vi "ActuatorSetup_HORNDOWN_1000.vi"() -> ()   [LabVIEW 2017]
uses:
  Generic_Common/WeldAutomation/Global_Variable_Status_Indicator.vi
panel:
  out "Pre part contanct in inch":dbl
  out "Pre Part Contanct distance in mm pre":dbl
  out "Absolute distance in inch":dbl
  out "Absolute distance in mm":dbl
  out "#Iterations:":dbl format="%-#1.6g"
  out "Welding Progress":u8(slide) scale=0.0..100.0
  out "Test Result":picture
  out "Performance Graph":cluster{dbl, u32}[](graph)
  # "Instructions:\n1. Make sure Ethernet cable from SC board connected to Laptop, \n2. Type netstat in command pompt to cross verify, SC port connection is established \n3. Then run the VI, press palm button first time button for actuator setup FPC will be perfomed\n4. Again press palm button to perform welding, second time onward welding will be perfomed\n5, To edit local_config.ini file to change the recipe parameters."
  # "Test execution sequence : \n1. Read SC, PC_AC parameters from INI file\n2. Send command to BL\n    a. MessageID_SC + Length (SC parameters) + SC parameters\n      b. MessageID_PC_AC  + Length (PC_AC parameters) + PC_AC parameters\n3. Receive response from BL after sending recipe parameters\n      c. ResponseID + Message \n4. Press palm button using USB6008 device\n5. Report Generation and Log generation"
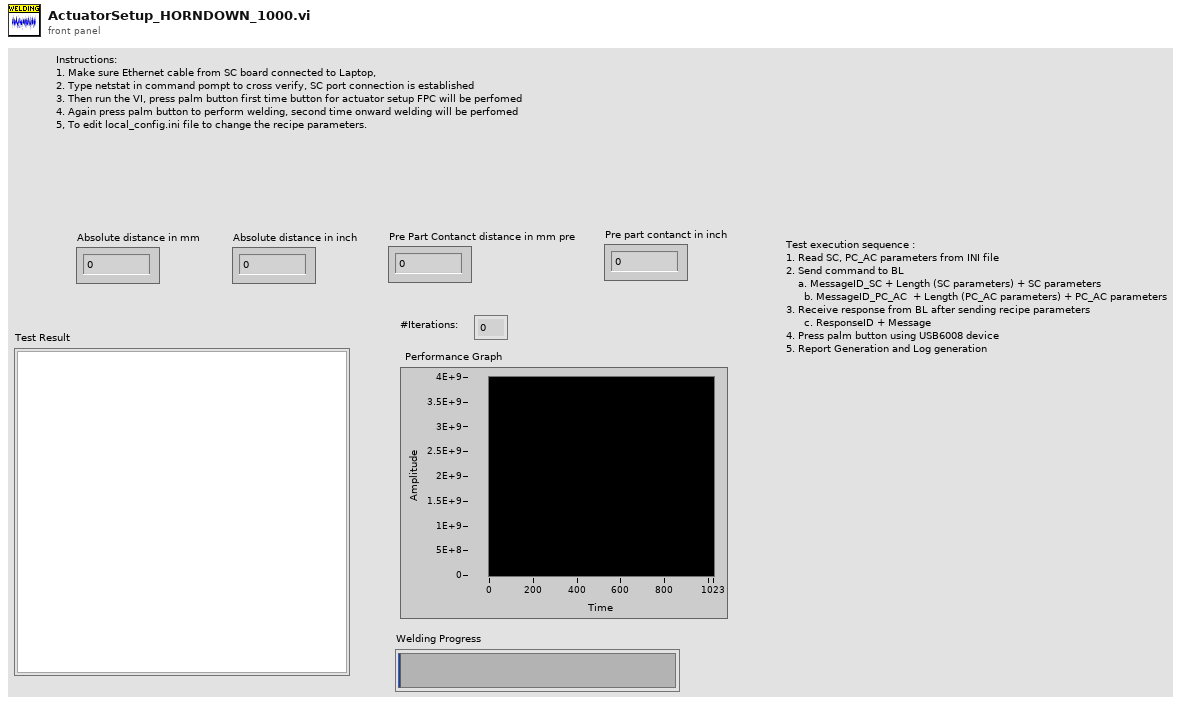
[diagram p1: front panel]
types:
  T1 = enum16{"open", "replace", "create", "open or create", "replace or create", "replace or create with confirmation"}
  T2 = cluster{"[0]":string, "[1]":string, "[2]":string, "[3]":string, "[4]":string, "[5]":string, "[6]":string, "[7]":string, "[8]":string}
  T3 = cluster{"Socket_IP_Address":string, "Socket_Port_Number":u16, "Global_ReportPath":path}
  T4 = cluster{"Iterations":u64, "DelayBetweenIterations":u32, "Time out":u32, "Message ID":i32, "Message Lenght":i32, "Response ID":i32, "Type of operation":i32, "Time stamp":string, "Test suite":string, "Report Path":path, "FW Version Path":path}
  T5 = typedef "imagedata.ctl" = cluster{"image type":i32, "image depth":i32, "image":u8[], "mask":u8[], "colors":u32[], "Rectangle":cluster{"left":i16, "top":i16, "right":i16, "bottom":i16}}
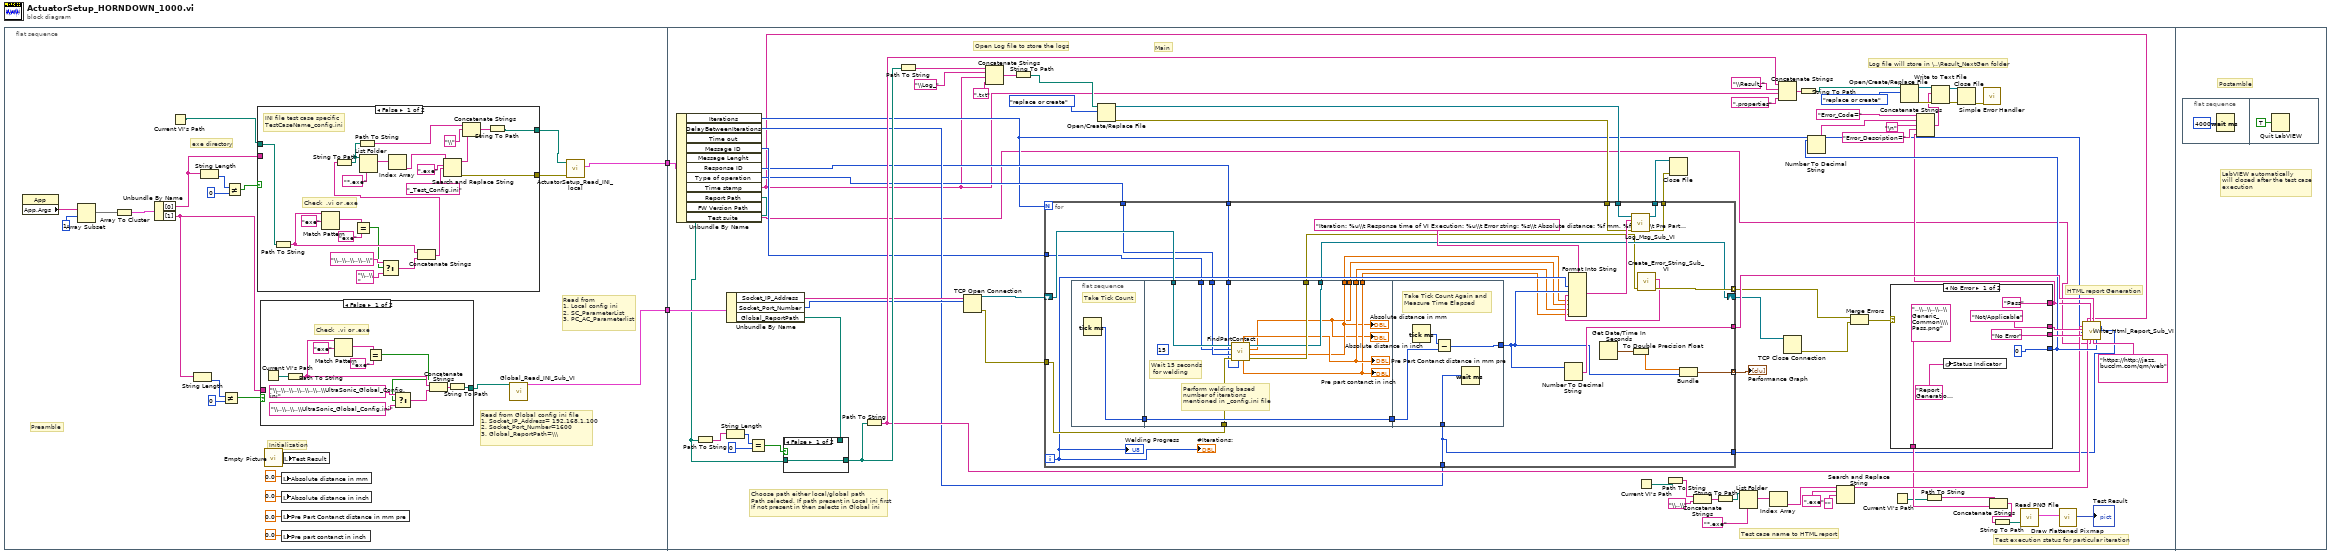
[diagram p0: block diagram]
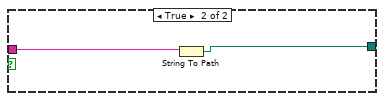
[diagram p2: hidden frame]
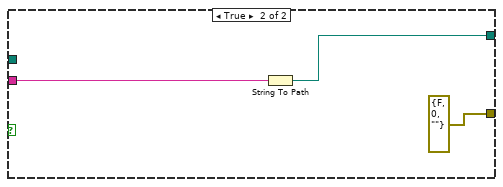
[diagram p3: hidden frame]
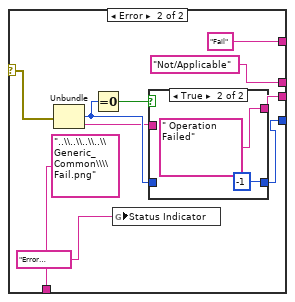
[diagram p5: hidden frame]
diagram:
  n1 = flat-sequence {
    tunnel: [w12] -> w2
    tunnel: [w8] -> w1
    tunnel: w2 -> [w86]
    tunnel: w1 -> [w71]
    frame #0 {
      # "Initialization"
      # "exe directory"
      # "Read from Global config ini file\n1. Socket_IP_Address= 192.168.1.100\n2. Socket_Port_Number=1600\n3. Global_ReportPath=\\\\\\"
      # "Read from\n1. Local config ini\n2. SC_ParameterList\n3. PC_AC_Parameterlist"
      # "Preamble"
      n2 = property class="App"() -> ("App.Args"=w14:string[])  [unwired: 2 in, 2 out]
      n3 = Array Subset "Array Subset"(array=w14, index=1) -> (w15:string[])  [unwired: 1 in]
      n4 = Array To Cluster(array=w15) -> (cluster=w16:T2)
      n5 = Unbundle By Name "Unbundle By Name"(w16) -> ("[0]"=w20:string, "[1]"=w23:string)
      n6 = Current VI's Path() -> (path=w11:path)
      n7 = String Length(string=w23) -> (length=w24:i32)
      n8 = String Length(string=w20) -> (length=w17:i32)
      n9 = Not Equal?(x=w24, y=0) -> (x != y?=w22:bool)
      n10 = Not Equal?(x=w17, y=0) -> (x != y?=w19:bool)
      n11 = case shown="False" w19 {
        tunnel: w20 -> [_ w63]
        tunnel: [w52 w62] -> w10
        tunnel: [w51 errorcluster {"status"=FALSE, "code"=0, "source"=""} ("error out")] -> w9
        tunnel: w11 -> [w40 _]
        frame False {
          # "Check  .vi or .exe"
          # "INI file test case specific\nTestCaseName_config.ini"
          n12 = Path To String(path=w40) -> (string=w45:string)
          n13 = Match Pattern(string=w45, regular expression="exe") -> (match substring=w44:string)  [unwired: 1 in, 3 out]
          n14 = Equal?(x=w44, y="exe") -> (x = y?=w42:bool)
          n15 = Select(t="\\..\\..\\..\\..\\" ("string"), s=w42, f="\\..\\" ("string")) -> (s? t:f=w46:string)
          n16 = Concatenate Strings(w45, w46) -> (w39:string)
          n17 = String To Path(string=w39) -> (path=w50:path)
          n18 = Path To String(path=w50) -> (string=w49:string)
          n19 = List Folder(path=w50, pattern="*.exe") -> (filenames=w54:string[])  [unwired: 2 in, 3 out]
          n20 = Index Array(array=w54) -> (element=w53:string)  [unwired: 1 in]
          n21 = Search and Replace String(input string=w53, search string=".exe", replace string="_Test_Config.ini" ("replace string (\"\")")) -> (result string=w58:string, error out=w51:errorcluster)  [unwired: 5 in, 2 out]
          n22 = Concatenate Strings(w49, "\\" ("string"), w58) -> (w56:string)
          n23 = String To Path(string=w56) -> (path=w52:path)
        }
        frame True {
          n24 = String To Path(string=w63) -> (path=w62:path)
        }
      }
      n25 = case shown="False" w22 {
        tunnel: [w35 w38] -> w25
        tunnel: w23 -> [_ w37]
        frame False {
          # "Check  .vi or .exe"
          n26 = Current VI's Path() -> (path=w27:path)
          n27 = Path To String(path=w27) -> (string=w31:string)
          n28 = Match Pattern(string=w31, regular expression="exe") -> (match substring=w30:string)  [unwired: 1 in, 3 out]
          n29 = Equal?(x=w30, y="exe") -> (x = y?=w28:bool)
          n30 = Select(t="\\..\\..\\..\\..\\..\\..\\UltraSonic_Global_Config.ini" ("string"), s=w28, f="\\..\\..\\..\\UltraSonic_Global_Config.ini" ("string")) -> (s? t:f=w32:string)
          n31 = Concatenate Strings(w31, w32) -> (w36:string)
          n32 = String To Path(string=w36) -> (path=w35:path)
        }
        frame True {
          n33 = String To Path(string=w37) -> (path=w38:path)
        }
      }
      n34 = call "Empty Picture"() -> ("empty picture"=w3:picture)
      n35 = local write "Absolute distance in mm"(0.0) -> ()
      n36 = local write "Absolute distance in inch"(0.0) -> ()
      n37 = local write "Pre Part Contanct distance in mm pre"(0.0) -> ()
      n38 = local write "Pre part contanct in inch"(0.0) -> ()
      n39 = local write "Test Result"(w3) -> ()
      n40 = call "Global_Read_INI_Sub_VI.vi"("Config File Path"=w25) -> ("output cluster"=w12:T3)  [unwired: 14 in]
      n41 = call "ActuatorSetup_Read_INI_local.vi"("Error In"=w9, "Config File Path"=w10) -> ("Actuator setup Parameters"=w8:T4)  [unwired: 8 in, 1 out]
    }
    frame #1 {
      # "Open Log file to store the logs"
      # "HTML report Generation"
      # "Log file will store in \\..\\Result_NextGen folder"
      # "Test execution status for particular iteration"
      # "Test case name to HTML report"
      # "Choose path either local/global path\nPath selected, If path present in Local ini first\nIf not present in then selects in Global ini"
      # "Main"
      n42 = Unbundle By Name(w71) -> ("Iterations"=w67:u64, "DelayBetweenIterations"=w74:u32, "Message ID"=w70:i32, "Response ID"=w69:i32, "Type of operation"=w68:i32, "Time stamp"=w65:string, "Report Path"=w72:path, "Test suite"=w66:string)  [unwired: 3 out]
      n43 = Path To String(path=w72) -> (string=w73:string)
      n44 = String Length(string=w73) -> (length=w129:i32)
      n45 = Unbundle By Name(w86) -> ("Socket_IP_Address"=w83:string, "Socket_Port_Number"=w82:u16, "Global_ReportPath"=w85:path)
      n46 = Equal?(x=w129, y=0) -> (x = y?=w127:bool)
      n47 = case shown="False" w127 {
        tunnel: w85 -> [_ w141]
        tunnel: [w140 w141] -> w126
        tunnel: w72 -> [w140 _]
        frame False {
        }
        frame True {
        }
      }
      n48 = Path To String(path=w126) -> (string=w103:string)
      n49 = Path To String(path=w126) -> (string=w131:string)
      n50 = TCP Open Connection(address=w83, remote port or service name=w82) -> (connection ID=w79:refnum<k5>, error out=w81:errorcluster)  [unwired: 3 in]
      n51 = Concatenate Strings(w131, "\\Log_" ("string"), w65, ".txt" ("string")) -> (w134:string)
      n52 = String To Path(string=w134) -> (path=w133:path)
      n53 = Open/Create/Replace File(file path (use dialog)=w133, operation (0:open)=T1."replace or create") -> (refnum out=w104:refnum<file>, error out=w107:errorcluster)  [unwired: 1 in, 4 out]
      n54 = for {
        N: w67 -> [_]
        tunnel: [w168] -> w137
        tunnel: w104 -> [w162]
        tunnel: [w161] -> w106
        tunnel: [w159] -> w105
        tunnel: [w164] -> w135 mode=indexing
        tunnel: w107 -> [w160]
        tunnel: [w157] -> w102 mode=indexing
        tunnel: w81 -> [w155]
        shift-right: [w152] -> w80
        shift-left: w79 -> [w154]
        tunnel: w74 -> [w142]
        tunnel: w68 -> [w145]
        tunnel: w70 -> [w144]
        tunnel: w69 -> [w143]
        tunnel: [w142] -> w64
        i -> [w153]
        n55 = flat-sequence {
          tunnel: [w170] -> w169
          tunnel: [w182] -> w151
          tunnel: w169 -> [w182]
          tunnel: w155 -> [w180]
          tunnel: w154 -> [w181]
          tunnel: [w178] -> w152
          tunnel: [w179] -> w150
          tunnel: [w172] -> w149
          tunnel: [w171] -> w148
          tunnel: [w177] -> w147
          tunnel: [w176] -> w146
          tunnel: w145 -> [w175]
          tunnel: w144 -> [w174]
          tunnel: w143 -> [w173]
          tunnel: w151 -> [w186]
          tunnel: [w184] -> w158
          tunnel: w142 -> [w183]
          frame #0 {
            # "Take Tick Count"
            n56 = Tick Count (ms)() -> (millisecond timer value=w170:u32)
          }
          frame #1 {
            (unwired) 15
            # "Wait 15 seconds\n for welding"
            # "Perform welding based \nnumber of iterations\nmentioned in _config.ini file"
            n57 = call "FindPartContact.vi"("Response actuator"=w173, "Error In"=w180, "Type of operation"=w175, "Actuator command"=w174, "connection ID"=w181) -> ("Error Out"=w179:errorcluster, "Absolute distance mm"=w172:dbl, "Absolute distance inch"=w171:dbl, "connection ID out"=w178:refnum<k5>, "Pre Part contact inch"=w176:dbl, "Pre Part Contact mm"=w177:dbl)  [unwired: 1 in]
            "Absolute distance in mm" <- w172
            "Absolute distance in inch" <- w171
            "Pre Part Contanct distance in mm pre" <- w177
            "Pre part contanct in inch" <- w176
          }
          frame #2 {
            # "Take Tick Count Again and Measure Time Elapsed"
            n58 = Tick Count (ms)() -> (millisecond timer value=w185:u32)
            n59 = Subtract(x=w185, y=w186) -> (x-y=w184:u32)
            n60 = Wait (ms)(milliseconds to wait=w183) -> ()  [unwired: 1 out]
          }
        }
        n61 = Number To Decimal String(number=w158) -> (decimal integer string=w168:string)  [unwired: 1 in]
        n62 = Get Date/Time In Seconds() -> (seconds since 1Jan1904=w165:timestamp)
        n63 = To Double Precision Float(number=w165) -> (double precision float=w166:dbl)
        n64 = call "Create_Error_String_Sub_VI.vi"("error in"=w150) -> ("error out"=w157:errorcluster, "Error String"=w156:string)  [unwired: 9 in]
        n65 = Format Into String(format string="Iteration: %u\\t Response time of VI Execution: %u\\t Error string: %s\\t Absolute distance: %f mm, %f inch \\t Pre Part Contact: %f mm, %f inch", w153, w158, w156, w149, w148, w147, w146) -> (resulting string=w163:string)  [unwired: 2 in, 1 out]
        n66 = call "Log_Msg_Sub_VI.vi"("error in (no error)"=w160, "String"=w163, "Byte Stream File in"=w162) -> ("error out"=w159:errorcluster, "Byte Stream File out"=w161:refnum<file>)  [unwired: 7 in]
        n67 = Bundle "Bundle"(w166, w158) -> (w164:cluster{dbl, u32})  [unwired: 1 in]
        "Welding Progress" <- w153
        "#Iterations:" <- w153
      }
      "Performance Graph" <- w135
      n68 = Current VI's Path() -> (path=w75:path)
      n69 = Path To String(path=w75) -> (string=w99:string)
      n70 = Close File(refnum=w106, error in=w105) -> ()  [unwired: 2 out]
      n71 = Concatenate Strings(w99, "\\..\\" ("string")) -> (w97:string)
      n72 = String To Path(string=w97) -> (path=w101:path)
      n73 = List Folder(path=w101, pattern="*.exe") -> (filenames=w96:string[])  [unwired: 2 in, 3 out]
      n74 = Index Array(array=w96) -> (element=w92:string)  [unwired: 1 in]
      n75 = Concatenate Strings(w103, "\\Result_" ("string"), w65, ".properties" ("string")) -> (w124:string)
      n76 = TCP Close Connection(connection ID=w80) -> (error out=w78:errorcluster)  [unwired: 2 in, 1 out]
      n77 = String To Path(string=w124) -> (path=w116:path)
      n78 = Search and Replace String(input string=w92, search string=".exe", replace string="" ("replace string (\"\")")) -> (result string=w95:string)  [unwired: 5 in, 3 out]
      n79 = Merge Errors "Merge Errors"(w102, w78) -> (w84:errorcluster)
      n80 = case shown="No Error" w84 {
        selector: w84 -> [_ w193]
        tunnel: ["Pass" "Fail"] -> w108
        tunnel: [0 ("code") w197] -> w112
        tunnel: ["No Error" ("source") w198] -> w139
        tunnel: ["Not/Applicable" "Not/Applicable"] -> w138
        tunnel: ["..\\..\\..\\..\\Generic_Common\\\\Pass.png" ("string") "..\\..\\..\\..\\Generic_Common\\\\Fail.png" ("string")] -> w87
        frame No Error {
          n81 = global write "Global_Variable_Status_Indicator.vi" "Status Indicator"("Report Generation inprogress...!!!" ("Current status")) -> ()
        }
        frame Error {
          n82 = Unbundle(w193) -> ("code"=w199:i32, "source"=w195:string)  [unwired: 1 out]
          n83 = Equal To 0?(x=w199) -> (x = 0?=w196:bool)
          n84 = global write "Global_Variable_Status_Indicator.vi" "Status Indicator"("Error occurred, Report Generation inprogress...!!!" ("Current status")) -> ()
          n85 = case shown="True" w196 {
            tunnel: [w204 -1 ("code")] -> w197
            tunnel: [w203 " Operation Failed" ("source")] -> w198
            tunnel: w199 -> [w204 _]
            tunnel: w195 -> [w203 _]
            frame False {
            }
            frame True {
            }
          }
        }
      }
      n86 = Number To Decimal String(number=w112) -> (decimal integer string=w111:string)  [unwired: 1 in]
      n87 = Current VI's Path() -> (path=w77:path)
      n88 = Open/Create/Replace File(file path (use dialog)=w116, operation (0:open)=T1."replace or create") -> (refnum out=w115:refnum<file>, error out=w120:errorcluster)  [unwired: 4 in, 1 out]
      n89 = Concatenate Strings("Error_Code=" ("string"), w111, "\n", "Error_Description=" ("string"), w108) -> (w114:string)
      n90 = Path To String(path=w77) -> (string=w76:string)
      n91 = Write to Text File(file (use dialog)=w115, text=w114, error in=w120) -> (refnum out=w119:refnum<file>, error out=w118:errorcluster)  [unwired: 1 in, 1 out]
      n92 = Close File(refnum=w119, error in=w118) -> (error out=w117:errorcluster)  [unwired: 1 out]
      n93 = call <vilib>:"Simple Error Handler.vi"("error in (no error)"=w117) -> ()  [unwired: 4 in, 5 out]
      n94 = Concatenate Strings(w76, w87) -> (w88:string)
      n95 = String To Path(string=w88) -> (path=w91:path)
      n96 = call <vilib>:"Read PNG File.vi"("path to PNG file"=w91) -> ("image data"=w89:T5)  [unwired: 8 in, 2 out]
      n97 = call <vilib>:"Draw Flattened Pixmap.vi"("image data"=w89) -> ("new picture"=→"Test Result":picture)  [unwired: 8 in]
      n98 = call "Write_Html_Report_Sub_VI.vi"("ReprtPath"=w103, "Remarks"=w138, "Iterations"=w67, "Error Description"=w139, "Timestamp"=w65, "TestCase"=w95, "Verdict"=w108, "TestSuite"=w66, "Time taken to execute  test in msec"=w137, "JazzDashboardLink"="https://http://jazz.bucclm.com/qm/web" ("TestSuite"), "Delay Between Iterations"=w64, "Error Code"=w112) -> ()  [unwired: 8 in]
    }
    frame #2 {
      # "LabVIEW automatically\nwill closed after the test case \nexecution"
      # "Postamble"
      n99 = flat-sequence {
        frame #0 {
          n100 = Wait (ms)(milliseconds to wait=u32 4000) -> ()  [unwired: 1 out]
        }
        frame #1 {
          n101 = Quit LabVIEW(quit? (T)=TRUE) -> ()
        }
      }
    }
  }
